vi "ZM_valve_state_VCH.vi"(9 "Parameters table MVCH":u32[](array[numeric])=[0, 0, 100, 100, 0, 300000, 60000, 100, 3], 10 "ZB01":bool, 11 "Z_In":T4={"Z_Source"=enum."local disabled", "Z_State"=enum."initialization", "ZM_State"=enum."initialization"}) -> (1 "t":u32, 3 "Z_Out":T4={"Z_Source"=enum."local disabled", "Z_State"=enum."initialization", "ZM_State"=enum."initialization"}, 4 "ZM_State_next":u32)   [LabVIEW 2019, in "Valves.lvlib"]
uses:
  Valves.lvlib
  Heating/ctl/Y_source.ctl
  ctl/Z_State_VCH.ctl
  ctl/ZM_State_VCH.ctl
  Trigers/RS.vi
  Timer Delay/Timer.vi
  Userlib.lvlib
  Heating/Heating.lvlib
panel:
  out "End":bool
  out "Stop":bool
  out "Start":bool
  # "T_valve_open_state"
  # "T_restart_delay"
  # "T_valve_open"
  # "T_valve_close"
  # "T_little_pause"
  # "T_start_delay"
  # "T_stop_delay"
  # "T_big_pause"
  # "N_repeat"
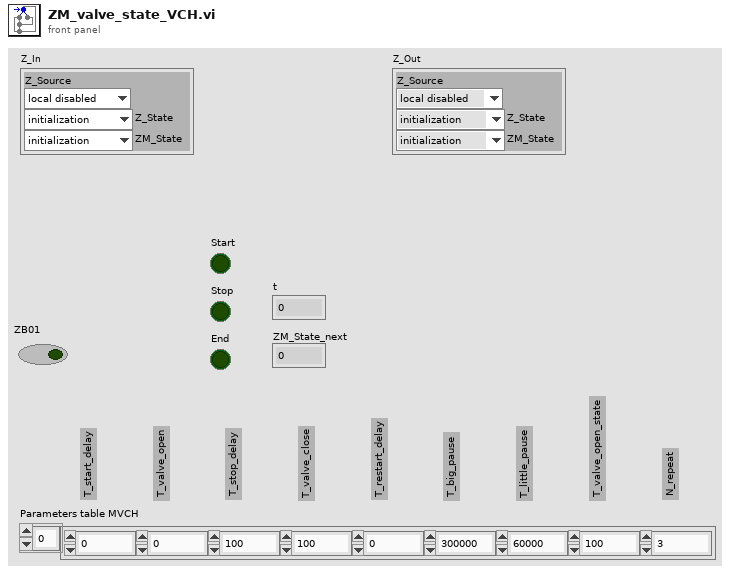
[diagram p1: front panel]
types:
  T1 = typedef "Heating.lvlib/Y_source.ctl" = enum8{"initialize", "local disabled", "local hand", "hand", "auto", "dist"}
  T2 = typedef "Valves.lvlib/Z_State_VCH.ctl" = enum8{"initialization", "alarm", "disabled", "not ready", "closed ready", "reserv", "reserv1", "reserv2", "reserv3", "check", "on min", "open", "on (closed)"}
  T3 = typedef "Valves.lvlib/ZM_State_VCH.ctl" = enum8{"initialization", "closed", "big_pause", "little_pause", "open", "close_cmd"}
  T4 = cluster{"Z_Source":T1, "Z_State":T2, "ZM_State":T3}
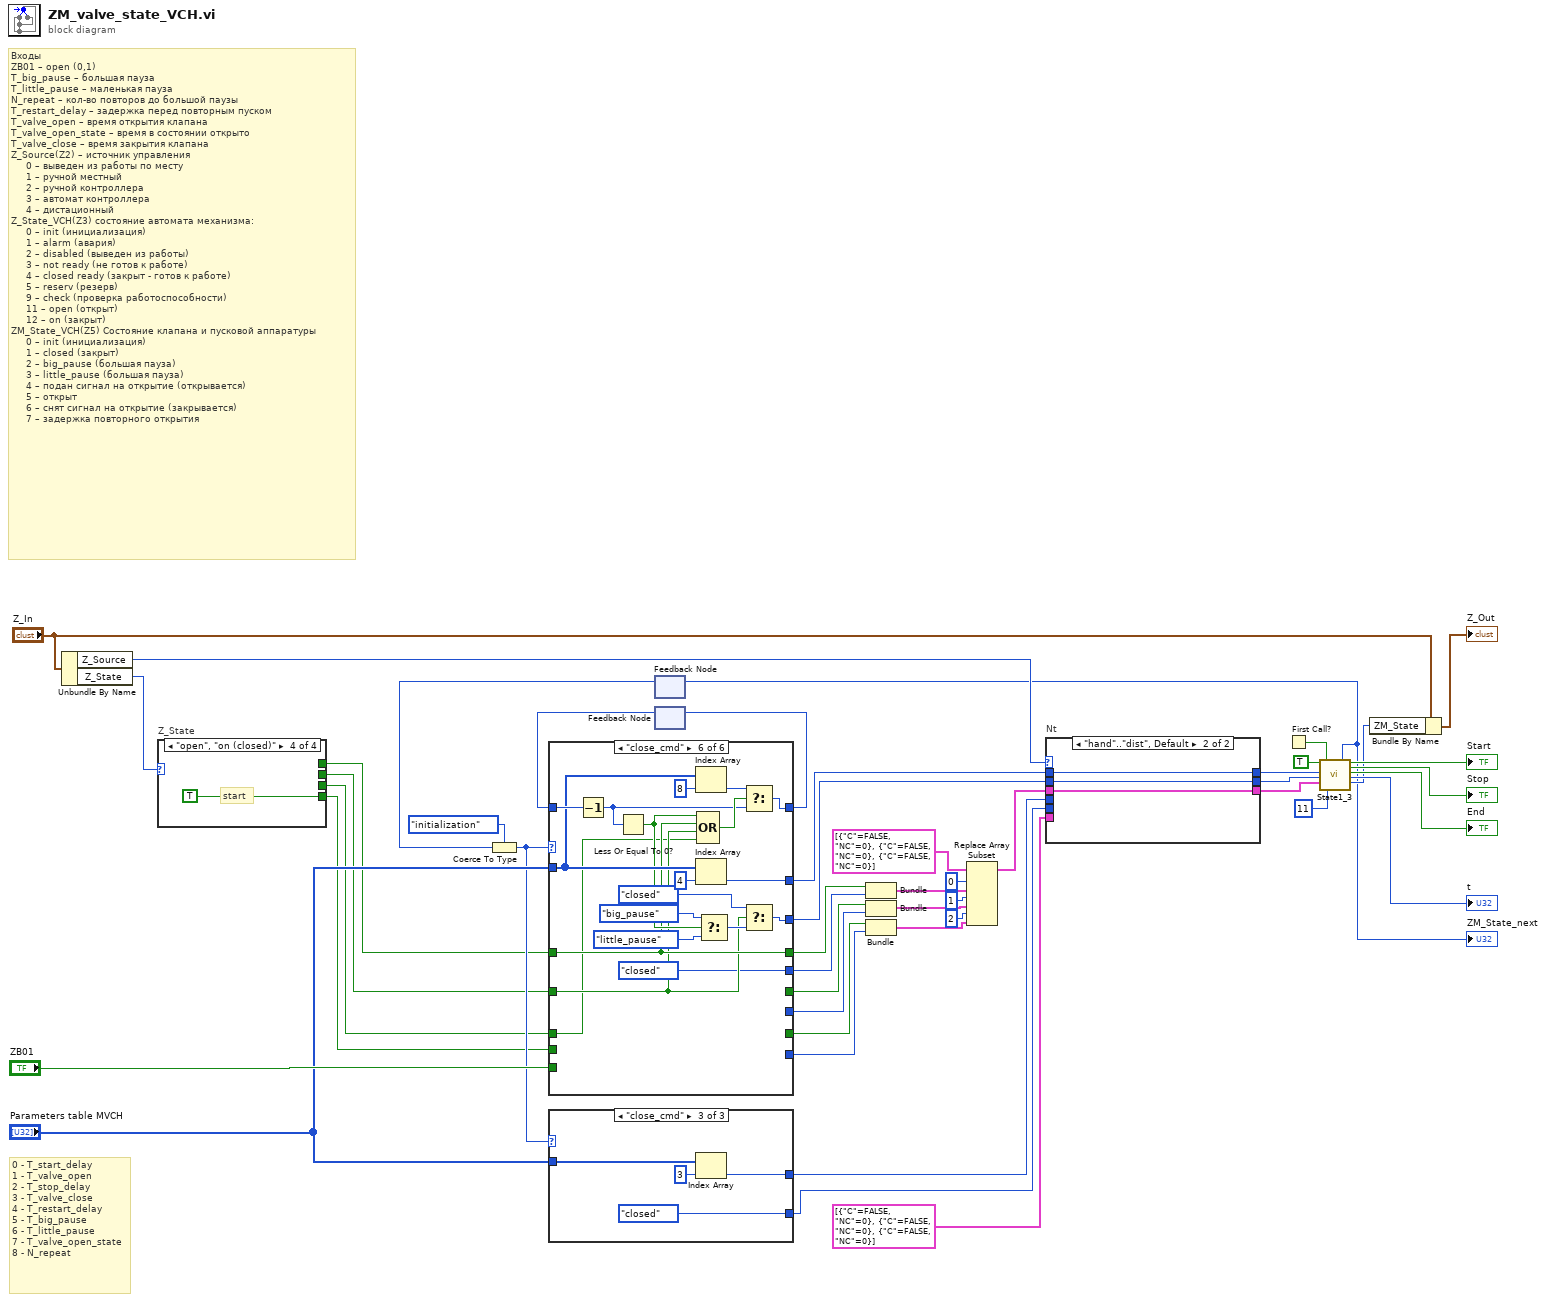
[diagram p0: block diagram]
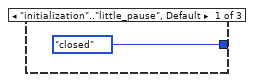
[diagram p3: hidden frame]
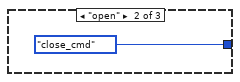
[diagram p4: hidden frame]
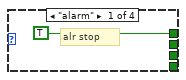
[diagram p5: hidden frame]
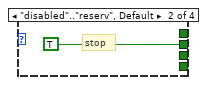
[diagram p6: hidden frame]
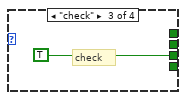
[diagram p7: hidden frame]
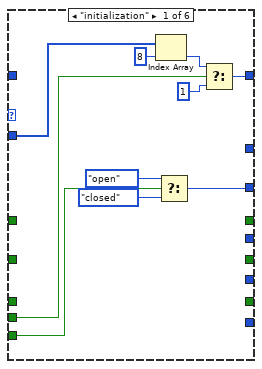
[diagram p8: hidden frame]
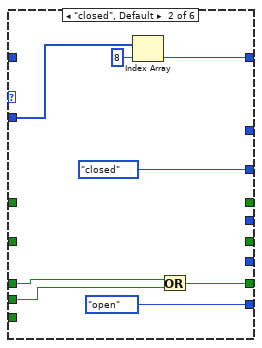
[diagram p9: hidden frame]
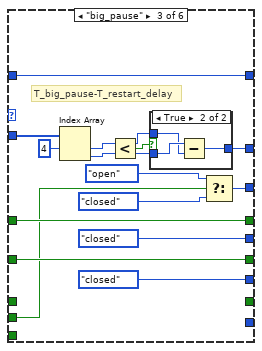
[diagram p10: hidden frame]
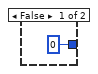
[diagram p11: hidden frame]
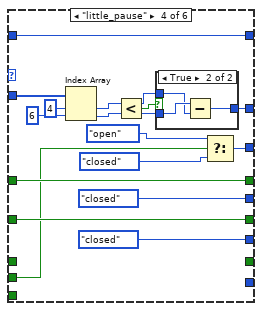
[diagram p12: hidden frame]
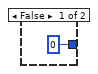
[diagram p13: hidden frame]
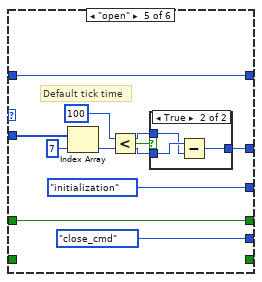
[diagram p14: hidden frame]
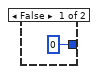
[diagram p15: hidden frame]
diagram:
  # "0 - T_start_delay\n1 - T_valve_open\n2 - T_stop_delay\n3 - T_valve_close\n4 - T_restart_delay\n5 - T_big_pause\n6 - T_little_pause\n7 - T_valve_open_state\n8 - N_repeat"
  # "Входы\nZB01 – open (0,1)\nT_big_pause – большая пауза\nT_little_pause – маленькая пауза\nN_repeat – кол-во повторов до большой паузы\nT_restart_delay – задержка перед повторным пуском\nT_valve_open – время открытия клапана\nT_valve_open_state – время в состоянии открыто\nT_valve_close – время закрытия клапана\nZ_Source(Z2) – источник управления\n     0 – выведен из работы по месту\n     1 – ручной местный\n     2 – ручной контроллера\n     3 – автомат контроллера\n     4 – дистационный\nZ_State_VCH(Z3) состояние автомата механизма:\n     0 – init (инициализация)\n     1 – alarm (авария)\n     2 – disabled (выведен из работы)\n     3 – not ready (не готов к работе)\n     4 – closed ready (закрыт - готов к работе)\n     5 – reserv (резерв)\n     9 – check (проверка работоспособности)\n     11 – open (открыт)\n     12 – on (закрыт)\nZM_State_VCH(Z5) Состояние клапана и пусковой аппаратуры\n     0 – init (инициализация)\n     1 – сlosed (закрыт)\n     2 – big_pause (большая пауза)\n     3 – little_pause (большая пауза)\n     4 – подан сигнал на открытие (открывается)\n     5 – открыт\n     6 – снят сигнал на открытие (закрывается)\n     7 – задержка повторного открытия"
  n1 = Unbundle By Name("Z_In") -> ("Z_Source"=w13:T1, "Z_State"=w12:T2)
  n2 = case "Z_State" shown="\"open\", \"on (closed)\"" w12 {
    tunnel: [_ TRUE _ _] -> w10
    tunnel: [_ _ TRUE _] -> w9
    tunnel: [TRUE _ _ _] -> w11
    tunnel: [_ _ _ TRUE] -> w8
    frame "alarm" {
      # "alr stop"
    }
    frame "disabled".."reserv", Default {
      # "stop"
    }
    frame "check" {
      # "check"
    }
    frame "open", "on (closed)" {
      # "start"
    }
  }
  n3 = feedback #1() -> (w40:u32)  [unwired: 1 in]
  n4 = Coerce To Type(0:w40, 1:ZM_State_VCH."initialization" ("ZM_State_VCH")) -> (2:w41:T3)
  n5 = case shown="\"close_cmd\"" w41 {
    tunnel: "Parameters table MVCH" -> [_ _ w54]
    tunnel: [ZM_State_VCH."closed" ("ZM_State_VCH") ZM_State_VCH."close_cmd" ("ZM_State_VCH") ZM_State_VCH."closed" ("ZM_State_VCH")] -> w5
    tunnel: [_ _ w55] -> w4
    frame "initialization".."little_pause", Default {
    }
    frame "open" {
    }
    frame "close_cmd" {
      n6 = Index Array(array=w54, index=3) -> (element=w55:u32)
    }
  }
  n7 = feedback #2() -> (w45:u32)  [unwired: 1 in]
  n8 = case shown="\"close_cmd\"" w41 {
    tunnel: "Parameters table MVCH" -> [w65 w68 w88 w99 w122 w140]
    tunnel: [w64 ZM_State_VCH."closed" ("ZM_State_VCH") w84 w96 ZM_State_VCH."initialization" ("ZM_State_VCH") w134] -> w6
    tunnel: [_ _ w75 w100 w114 w145] -> w1
    tunnel: [_ _ w86 w108 w120 w136] -> w17
    tunnel: [_ _ ZM_State_VCH."closed" ("ZM_State_VCH") ZM_State_VCH."closed" ("ZM_State_VCH") ZM_State_VCH."close_cmd" ("ZM_State_VCH") ZM_State_VCH."closed" ("ZM_State_VCH")] -> w18
    tunnel: [_ w73 _ _ _ _] -> w21
    tunnel: w9 -> [_ w74 _ _ _ w132]
    tunnel: [_ ZM_State_VCH."open" ("ZM_State_VCH") _ _ _ _] -> w22
    tunnel: w10 -> [_ _ w85 w107 _ w133]
    tunnel: [_ _ w85 w107 _ _] -> w19
    tunnel: [_ _ ZM_State_VCH."closed" ("ZM_State_VCH") ZM_State_VCH."closed" ("ZM_State_VCH") _ _] -> w20
    tunnel: w11 -> [_ _ w86 w108 w120 w136]
    tunnel: "ZB01" -> [w63 _ _ _ _ _]
    tunnel: [w62 w67 w87 w109 w121 w141] -> w46
    tunnel: w45 -> [_ _ w87 w109 w121 w142]
    tunnel: w8 -> [w59 w72 w83 w95 _ _]
    frame "initialization" {
      n9 = Index Array(array=w65, index=8) -> (element=w61:u32)
      n10 = Select(t=ZM_State_VCH."open" ("ZM_State_VCH"), s=w63, f=ZM_State_VCH."closed" ("ZM_State_VCH")) -> (s? t:f=w64:T3)
      n11 = Select(t=w61, s=w59, f=u32 1 ("End step")) -> (s? t:f=w62:u32)
    }
    frame "closed", Default {
      n12 = Index Array(array=w68, index=8) -> (element=w67:u32)
      n13 = Or(x=w74, y=w72) -> (x .or. y?=w73:bool)
    }
    frame "big_pause" {
      # "T_big_pause-T_restart_delay"
      n14 = Index Array(array=w88, index #1=4 ("index")) -> (element #1=w77:u32, element #2=w76:u32)  [unwired: 1 in]
      n15 = Less?(x=w77, y=w76) -> (x < y?=w78:bool)
      n16 = case shown="True" w78 {
        tunnel: w77 -> [_ w91]
        tunnel: w76 -> [_ w92]
        tunnel: [u32 0 w93] -> w75
        frame False {
        }
        frame True {
          n17 = Subtract(x=w92, y=w91) -> (x-y=w93:u32)
        }
      }
      n18 = Select(t=ZM_State_VCH."open" ("ZM_State_VCH"), s=w83, f=ZM_State_VCH."closed" ("ZM_State_VCH")) -> (s? t:f=w84:T3)
    }
    frame "little_pause" {
      n19 = Index Array(array=w99, index #1=4 ("index"), index #2=6 ("index")) -> (element #1=w102:u32, element #2=w101:u32)
      n20 = Less?(x=w102, y=w101) -> (x < y?=w103:bool)
      n21 = case shown="True" w103 {
        tunnel: w102 -> [_ w111]
        tunnel: w101 -> [_ w112]
        tunnel: [u32 0 w113] -> w100
        frame False {
        }
        frame True {
          n22 = Subtract(x=w112, y=w111) -> (x-y=w113:u32)
        }
      }
      n23 = Select(t=ZM_State_VCH."open" ("ZM_State_VCH"), s=w95, f=ZM_State_VCH."closed" ("ZM_State_VCH")) -> (s? t:f=w96:T3)
    }
    frame "open" {
      w115 = u32 100 ("element")
      # "Default tick time"
      n24 = Index Array(array=w122, index=7) -> (element=w116:u32)
      n25 = Less?(x=w115, y=w116) -> (x < y?=w117:bool)
      n26 = case shown="True" w117 {
        tunnel: w115 -> [_ w125]
        tunnel: w116 -> [_ w126]
        tunnel: [u32 0 w127] -> w114
        frame False {
        }
        frame True {
          n27 = Subtract(x=w126, y=w125) -> (x-y=w127:u32)
        }
      }
    }
    frame "close_cmd" {
      n28 = Decrement(x=w142) -> (x-1=w138:u32)
      n29 = Less Or Equal To 0?(x=w138) -> (x <= 0?=w137:bool)
      n30 = Index Array(array=w140, index=8) -> (element=w144:u32)
      n31 = Index Array(array=w140, index=4) -> (element=w145:u32)
      n32 = Compound Arithmetic op=OR(w137, w136, w133, w132) -> (w139:bool)
      n33 = Select(t=ZM_State_VCH."big_pause" ("ZM_State_VCH"), s=w137, f=ZM_State_VCH."little_pause" ("ZM_State_VCH")) -> (s? t:f=w135:T3)
      n34 = Select(t=w144, s=w139, f=w138) -> (s? t:f=w141:u32)
      n35 = Select(t=ZM_State_VCH."closed" ("ZM_State_VCH"), s=w133, f=w135) -> (s? t:f=w134:T3)
    }
  }
  n36 = feedback-in #2(w46) -> ()
  n37 = Bundle(w17, "ZM_State_VCH"=w18) -> (w34:cluster{bool, "ZM_State_VCH":T3})  [unwired: 1 in]
  n38 = Bundle(w19, "ZM_State_VCH"=w20) -> (w31:cluster{bool, "ZM_State_VCH":T3})  [unwired: 1 in]
  n39 = Bundle(w21, "ZM_State_VCH"=w22) -> (w30:cluster{bool, "ZM_State_VCH":T3})  [unwired: 1 in]
  n40 = Replace Array Subset(array=cluster{"C":bool, "NC":u32}[] [{"C"=FALSE, "NC"=0}, {"C"=FALSE, "NC"=0}, {"C"=FALSE, "NC"=0}] ("appended array"), new element #1=w34, index #1=0 ("index"), new element #2=w31, index #2=1 ("index"), new element #3=w30, index #3=2 ("index")) -> (w28:cluster{"C":bool, "NC":u32}[])
  n41 = case "Nt" shown="\"hand\"..\"dist\", Default" w13 {
    tunnel: w6 -> [_ w152]
    tunnel: w28 -> [_ w151]
    tunnel: [w148 w152] -> w29
    tunnel: [w149 w151] -> w27
    tunnel: w5 -> [w148 _]
    tunnel: cluster{"C":bool, "NC":u32}[] [{"C"=FALSE, "NC"=0}, {"C"=FALSE, "NC"=0}, {"C"=FALSE, "NC"=0}] ("appended array") -> [w149 _]
    tunnel: w4 -> [w147 _]
    tunnel: [w147 w150] -> w3
    tunnel: w1 -> [_ w150]
    frame "local disabled", "local hand" {
    }
    frame "hand".."dist", Default {
    }
  }
  n42 = First Call?() -> (First Call?: T/F=w38:bool)
  n43 = call "State1_3.vi"("Start"=TRUE, "t"=w3, "Nt"=w29, "C_table"=w27, "Reset"=w38, "End step"=u32 11) -> ("N next"=w2:u32, "Start"=→"Start":bool, "Stop"=→"Stop":bool, "End"=→"End":bool, "t"=→"t":u32, "N curr"=w15:u32)  [unwired: 8 in]
  "ZM_State_next" <- w2
  n44 = feedback-in #1(w2) -> ()
  n45 = Bundle By Name(cluster="Z_In", "ZM_State"=w15) -> (→"Z_Out":T4)
